vi "test_sort_nodes.vi"() -> ()   [LabVIEW 2020]
uses:
  api/Node/Node.lvclass
  api/DiGraph/DiGraph.lvclass
  C:/Projects/labview-project-load-tools/source/submodules/graph-api-labview/source/api/Graph/Graph.lvclass
  api/Node/Node.lvclass/Node.ctl
  api/Graph/Graph.lvclass
panel:
  out "cycle detected":bool
  out "Array":string[](array[string])
  out "x = y?":bool[](array[boolean])
  out "nodes (sorted)":refnum<class "Node.lvclass">[](array[class])
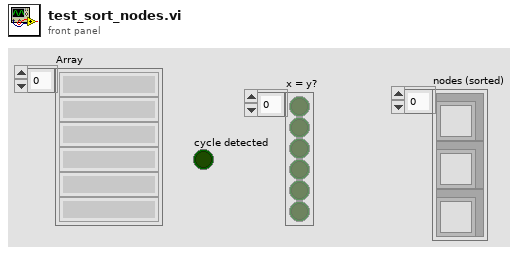
[diagram p1: front panel]
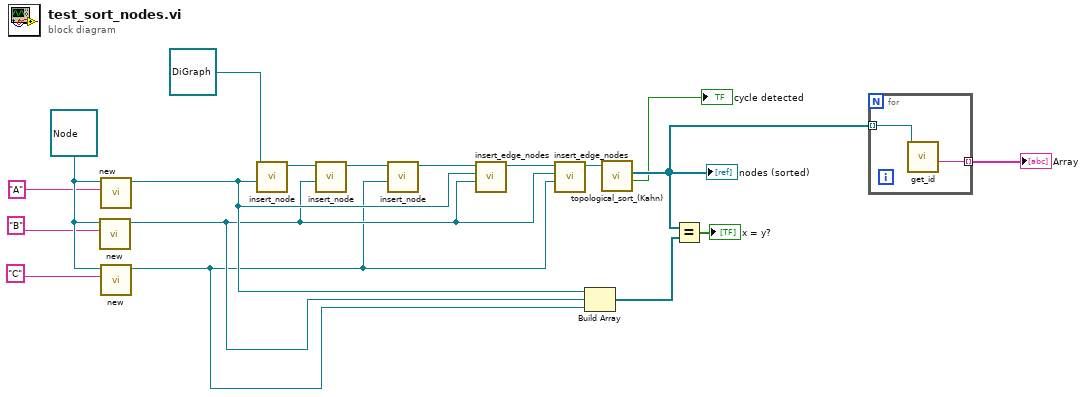
[diagram p0: block diagram]
diagram:
  w10 = refnum<class "Node.lvclass"> refnum ("Node in")
  n1 = call "new.vi"("label (\"\")"="B" ("label (\"\")"), "Node in"=w10) -> ("Node out"=w3:refnum<class "Node.lvclass">)  [unwired: 8 in, 1 out]
  n2 = call "new.vi"("label (\"\")"="A" ("label (\"\")"), "Node in"=w10) -> ("Node out"=w4:refnum<class "Node.lvclass">)  [unwired: 8 in, 1 out]
  n3 = call "new.vi"("label (\"\")"="C" ("label (\"\")"), "Node in"=w10) -> ("Node out"=w2:refnum<class "Node.lvclass">)  [unwired: 8 in, 1 out]
  n4 = call "insert_node.vi"("node"=w4, "graph"=refnum<class "DiGraph.lvclass"> refnum ("graph.lvlib:DiGraph.lvclass")) -> ("graph out"=w17:refnum<class "DiGraph.lvclass">)  [unwired: 7 in, 2 out]
  n5 = call "insert_node.vi"("node"=w3, "graph"=w17) -> ("graph out"=w16:refnum<class "DiGraph.lvclass">)  [unwired: 7 in, 2 out]
  n6 = call "insert_node.vi"("node"=w2, "graph"=w16) -> ("graph out"=w15:refnum<class "DiGraph.lvclass">)  [unwired: 7 in, 2 out]
  n7 = call-dynamic "insert_edge_nodes.vi"("node-b"=w3, "node-a"=w4, "graph"=w15) -> ("graph out"=w14:refnum<class "DiGraph.lvclass">)  [unwired: 5 in, 3 out]
  n8 = call-dynamic "insert_edge_nodes.vi"("node-b"=w2, "node-a"=w3, "graph"=w14) -> ("graph out"=w13:refnum<class "DiGraph.lvclass">)  [unwired: 5 in, 3 out]
  n9 = Build Array(w4, w3, w2) -> (w12:refnum<class "Node.lvclass">[])
  n10 = call "topological_sort_(Kahn).vi"("DiGraph in"=w13) -> ("cycle detected"=→"cycle detected":bool, "nodes (sorted)"=w6:refnum<class "Node.lvclass">[])  [unwired: 8 in, 1 out]
  "nodes (sorted)" <- w6
  n11 = Equal?(x=w6, y=w12) -> (x = y?=→"x = y?":bool[])
  n12 = for {
    tunnel: w6 -> [w20] mode=indexing
    tunnel: [w19] -> w5 mode=indexing
    n13 = call "get_id.vi"("node"=w20) -> ("label"=w19:string)  [unwired: 9 in, 1 out]
  }
  "Array" <- w5
